vi "getSessionKey.vi"(8 "error in (no error)":errorcluster, 11 "Experiment in":refnum<class "Experiment.lvclass">) -> (0 "error out":errorcluster, 2 "Session Key":cluster{"session":dbl, "animal_id":dbl}, 3 "Experiment out":refnum<class "Experiment.lvclass">)   [LabVIEW 2014, in "Experiment.lvclass"]
uses:
  Experiment.lvclass
  Experiment.lvclass/Experiment.ctl
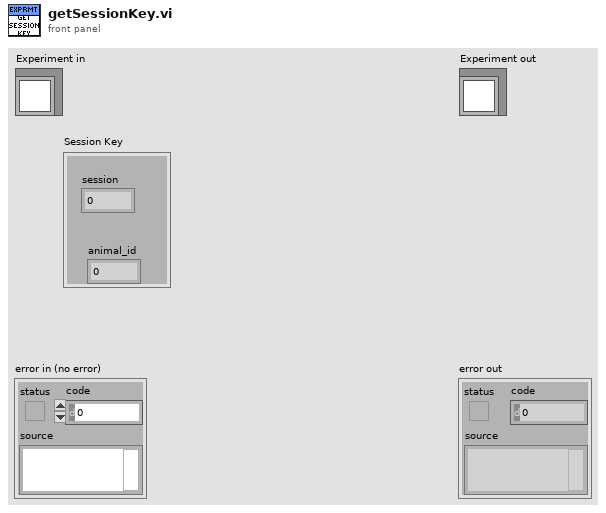
[diagram p1: front panel]
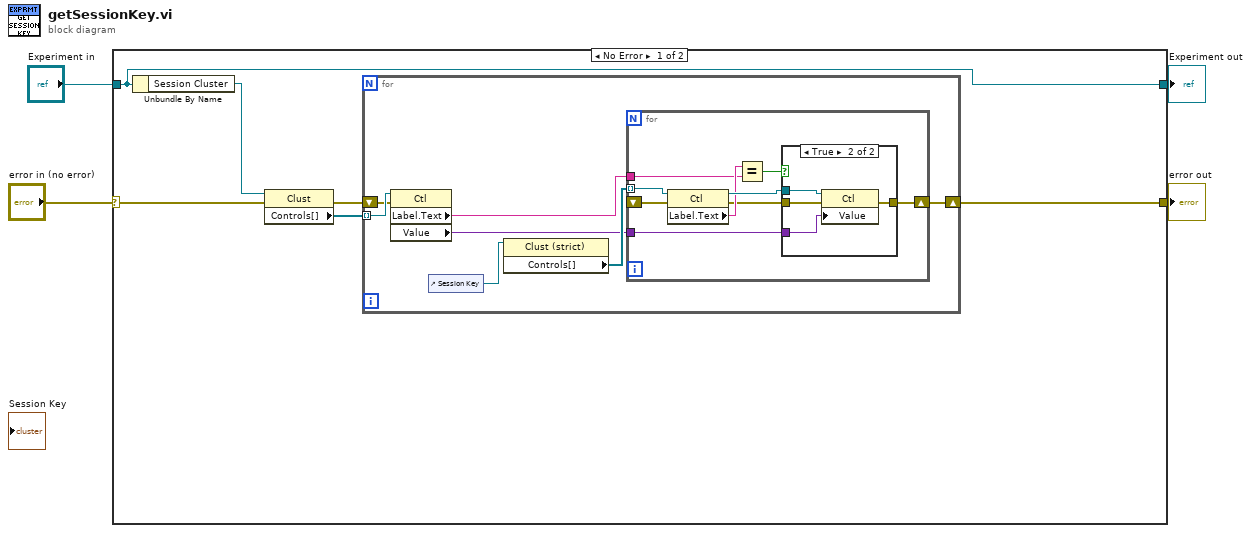
[diagram p0: block diagram]
diagram:
  n1 = case shown="No Error" "error in (no error)" {
    selector: "error in (no error)" -> [w7 w33]
    tunnel: [w5 w33] -> w3
    tunnel: [w10 w32] -> w1
    tunnel: "Experiment in" -> [w10 w32]
    frame No Error {
      n2 = Unbundle By Name(w10) -> ("Session Cluster"=w8:refnum<vi>)
      n3 = property class="Clust"(reference=w8, error in=w7) -> (error out=w6:errorcluster, "Controls[]"=w9:refnum<vi>[])  [unwired: 1 out]
      n4 = for {
        tunnel: w9 -> [w17] mode=indexing
        shift-right: [w11] -> w5
        shift-left: w6 -> [w16]
        n5 = property class="Ctl"(reference=w17, error in=w16) -> ("Label.Text"=w13:string, "Value"=w12:variant)  [unwired: 2 out]
        n6 = control-ref of="Session Key"() -> (w14:refnum<vi>)
        n7 = property class="Clust (strict)"(reference=w14) -> ("Controls[]"=w15:refnum<vi>[])  [unwired: 1 in, 2 out]
        n8 = for {
          tunnel: w15 -> [w26] mode=indexing
          shift-right: [w20] -> w11
          shift-left: _ -> [w22]
          tunnel: w13 -> [w19]
          tunnel: w12 -> [w18]
          n9 = property class="Ctl"(reference=w26, error in=w22) -> (reference out=w25:refnum<vi>, error out=w21:errorcluster, "Label.Text"=w23:string)
          n10 = Equal?(x=w23, y=w19) -> (x = y?=w24:bool)
          n11 = case shown="True" w24 {
            tunnel: w25 -> [_ w31]
            tunnel: w21 -> [w27 w30]
            tunnel: [w27 w29] -> w20
            tunnel: w18 -> [_ w28]
            frame False {
            }
            frame True {
              n12 = property class="Ctl"(reference=w31, error in=w30, "Value"=w28) -> (error out=w29:errorcluster)  [unwired: 1 out]
            }
          }
        }
      }
    }
    frame Error {
    }
  }
  "error out" <- w3
  "Experiment out" <- w1
